vi "find_corner.vi"(11 "XY in":dbl[][](array[numeric])) -> (2 "left top":dbl[](array[numeric]), 3 "right bottom":dbl[](array[numeric]))   [LabVIEW 2017]
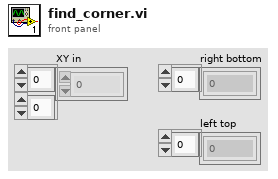
[diagram p1: front panel]
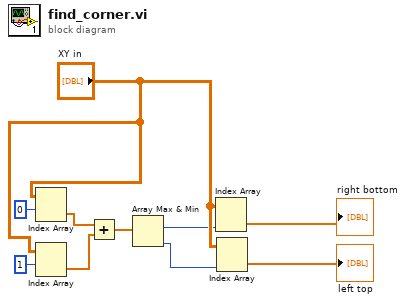
[diagram p0: block diagram]
diagram:
  n1 = Index Array "Index Array"(array="XY in", index (row)=0) -> (element=w3:dbl[])  [unwired: 1 in]
  n2 = Index Array(array="XY in", index (row)=1) -> (element=w4:dbl[])  [unwired: 1 in]
  n3 = Add(x=w3, y=w4) -> (x+y=w5:dbl[])
  n4 = Array Max & Min(array=w5) -> (max index (indices)=w7:i32, min index (indices)=w8:i32)  [unwired: 2 out]
  n5 = Index Array "Index Array"(array="XY in", index (col)=w7) -> (element=→"right bottom":dbl[])  [unwired: 1 in]
  n6 = Index Array "Index Array"(array="XY in", index (col)=w8) -> (element=→"left top":dbl[])  [unwired: 1 in]
